vi "POSITION CONTROL.vi"(2 "Result":dbl, 8 "Goal":string, 11 "Current Color":string) -> ()   [LabVIEW 2019]
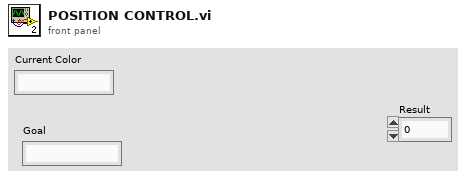
[diagram p1: front panel]
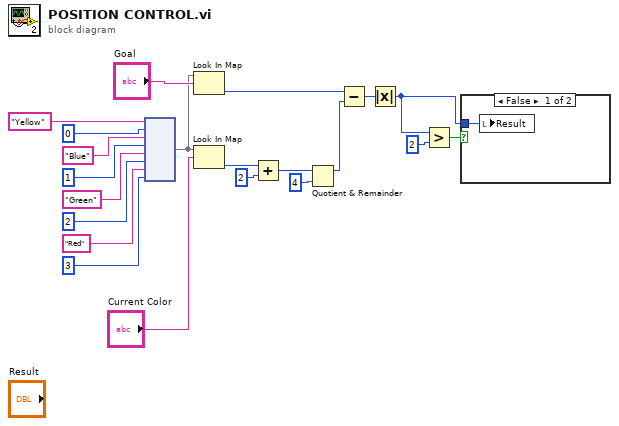
[diagram p0: block diagram]
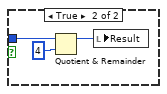
[diagram p2: hidden frame]
diagram:
  n1 = node("Yellow" ("key"), 0 ("value"), "Blue" ("key"), 1 ("value"), "Green" ("key"), 2 ("value"), "Red" ("key"), 3 ("value")) -> (w7:map{string, i32})
  n2 = Look In Map(map=w7, key="Goal") -> (value=w6:i32)  [unwired: 1 in, 1 out]
  n3 = Look In Map(map=w7, key="Current Color") -> (value=w12:i32)  [unwired: 1 in, 1 out]
  n4 = Add(x=w12, y=2) -> (x+y=w10:i32)
  n5 = Quotient & Remainder(x=w10, y=4) -> (x-y*floor(x/y)=w5:i32)  [unwired: 1 out]
  n6 = Subtract(x=w6, y=w5) -> (x-y=w4:i32)
  n7 = Absolute Value(x=w4) -> (abs(x)=w1:i32)
  n8 = Greater?(x=w1, y=2) -> (0:w2:bool)
  n9 = case shown="False" w2 {
    tunnel: w1 -> [w22 w25]
    frame False {
      n10 = local write "Result"(w22) -> ()
    }
    frame True {
      n11 = Quotient & Remainder(x=w25, y=4) -> (x-y*floor(x/y)=w23:i32)  [unwired: 1 out]
      n12 = local write "Result"(w23) -> ()
    }
  }
